vi "(DW7912)Update Wave Seq Value Ring.vi"(8 "error in (no error)":errorcluster caption="에러 입력(에러 없음)", 10 "Wave Seq Loop Ref In":refnum<vi>, 11 "Wave Seq Ref In":refnum<vi>) -> (0 "error out":errorcluster caption="에러 출력", 3 "index":u8)   [LabVIEW 2020]
uses:
  5ce0b5f2-788c-416b-a0e6-d14d701acb94.vi
  <vilib>/Comparison/Equal/Equal Functor/Equal Functor.lvclass
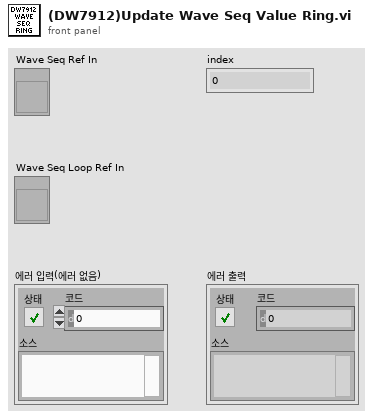
[diagram p1: front panel]
types:
  T1 = typedef "(Ctrl)DW7912_Wave Seq.ctl" = cluster{"Mode":u8, "Seq/Delay":u8}
  T2 = enum8{"Enabled", "Disabled", "Disabled and Grayed Out"}
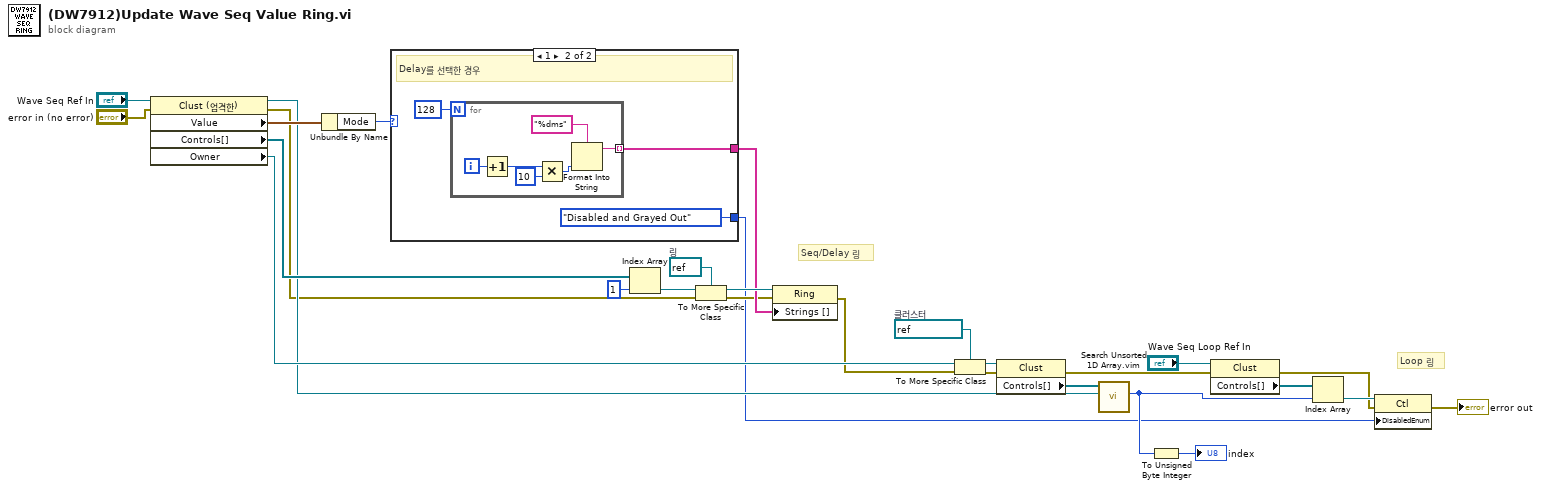
[diagram p0: block diagram]
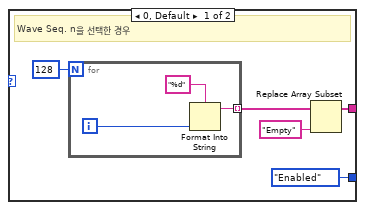
[diagram p2: hidden frame]
diagram:
  w17 = refnum<vi> refnum  # 클러스터
  w24 = refnum<vi> refnum  # 링
  # "Loop 링"
  # "Seq/Delay 링"
  n1 = property class="Clust (엄격한)"(reference="Wave Seq Ref In", error in="error in (no error)") -> (reference out=w10:refnum<vi>, error out=w6:errorcluster, "Value"=w12:T1, "Controls[]"=w27:refnum<vi>[], "Owner"=w11:refnum<vi>)
  n2 = Unbundle By Name(w12) -> ("Mode"=w20:u8)
  n3 = case shown="1" w20 {
    tunnel: [w31 w38] -> w23
    tunnel: [T2."Enabled" ("비활성화") T2."Disabled and Grayed Out" ("비활성화")] -> w2
    frame 0, Default {
      # "Wave Seq. n을 선택한 경우"
      n4 = for {
        N: 128 -> [_]
        tunnel: [w36] -> w32 mode=indexing
        i -> [w34]
        n5 = Format Into String(format string="%d" ("포맷 문자열"), w34) -> (resulting string=w36:string)  [unwired: 2 in, 1 out]
      }
      n6 = Replace Array Subset(array=w32, new element="Empty" ("새 원소/부분배열")) -> (w31:string[])  [unwired: 1 in]
    }
    frame 1 {
      # "Delay를 선택한 경우"
      n7 = for {
        N: 128 -> [_]
        tunnel: [w44] -> w38 mode=indexing
        i -> [w45]
        n8 = Increment(x=w45) -> (x+1=w42:i32)
        n9 = Multiply(x=w42, y=10) -> (x*y=w41:i32)
        n10 = Format Into String(format string="%dms" ("포맷 문자열"), w41) -> (resulting string=w44:string)  [unwired: 2 in, 1 out]
      }
    }
  }
  n11 = Index Array(array=w27, index=1 ("인덱스")) -> (element=w26:refnum<vi>)
  n12 = To More Specific Class(target class=w24, reference=w26, error in=w6) -> (specific class reference=w25:refnum<vi>, error out=w22:errorcluster)
  n13 = property class="Ring"(reference=w25, error in=w22, "Strings []"=w23) -> (error out=w5:errorcluster)  [unwired: 1 out]
  n14 = To More Specific Class(target class=w17, reference=w11, error in=w5) -> (specific class reference=w18:refnum<vi>, error out=w9:errorcluster)
  n15 = property class="Clust"(reference=w18, error in=w9) -> (error out=w7:errorcluster, "Controls[]"=w16:refnum<vi>[])  [unwired: 1 out]
  n16 = call "Search Unsorted 1D Array.vim"("element"=w10, "unsorted 1D array"=w16) -> ("index of element"=w8:i32)  [unwired: 9 in]
  n17 = To Unsigned Byte Integer(number=w8) -> (unsigned 8bit integer=→"index":u8)
  n18 = property class="Clust"(reference="Wave Seq Loop Ref In", error in=w7) -> (error out=w4:errorcluster, "Controls[]"=w14:refnum<vi>[])  [unwired: 1 out]
  n19 = Index Array(array=w14, index=w8) -> (element=w13:refnum<vi>)
  n20 = property class="Ctl"(reference=w13, error in=w4, "DisabledEnum"=w2) -> (error out=→"error out":errorcluster)  [unwired: 1 out]
